vi "Get Object Item by Name.vi"(8 "error in (no error)":errorcluster, 10 "name":string, 11 "JSON Value In":refnum<class "JSON Value.lvclass">) -> (0 "error out":errorcluster, 1 "found":bool, 2 "Value":refnum<class "JSON Value.lvclass">, 3 "JSON Value Out":refnum<class "JSON Value.lvclass">)   [LabVIEW 2011, in "JSON Value.lvclass"]
doc: "Gets an object from a JSON collection by it's name.\n\nCopyright 2012 James David Powell, Shaun Rumbell and Ton Plomp\nMore information on http://lavag.org/topic/16217-cr-json-labview"
uses:
  JSON Value.lvclass
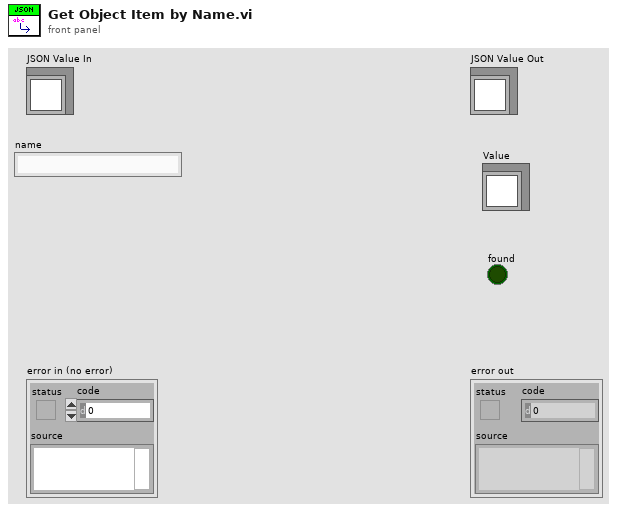
[diagram p1: front panel]
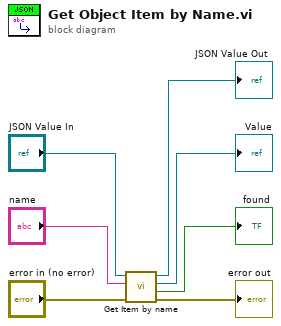
[diagram p0: block diagram]
diagram:
  n1 = call-dynamic "Get Item by name.vi"("error in (no error)"="error in (no error)", "name"="name", "JSON Value In"="JSON Value In") -> ("error out"=→"error out":errorcluster, "found"=→"found":bool, "Value"=→"Value":refnum<class "JSON Value.lvclass">, "JSON Value Out"=→"JSON Value Out":refnum<class "JSON Value.lvclass">)  [unwired: 5 in]
